vi "ReactionWheel.vi"(10 "Roll bias (deg)":dbl=0.5) -> ()   [LabVIEW 2021]
doc: "The myRIO Project template acquires acceleration data from the onboard accelerometer and displays the changes of acceleration values in a waveform chart."
uses:
  <vilib>/Platform/TimedLoop/XDataNode/timing_clust.ctl
  <vilib>/Platform/TimedLoop/XDataNode/nitl_modes.ctl
  <vilib>/Platform/TimedLoop/XDataNode/wakeup.ctl
  <vilib>/myRIO/Instrument Drivers/Onboard IO/PWM/typedefs/PWM Reference.ctl
  <vilib>/myRIO/Common/Instrument Driver Framework/Utilities/typedefs/myRIO Generic Hardware Reference.ctl
  <vilib>/myRIO/Common/Instrument Driver Framework/Utilities/typedefs/Hardware Version Enum.ctl
  <vilib>/myRIO/Common/Instrument Driver Framework/Utilities/typedefs/myRIO v1.0 Reference.ctl
  <vilib>/myRIO/Common/Instrument Driver Framework/Utilities/typedefs/Generic FPGA Reference.ctl
  <vilib>/myRIO/Common/Instrument Driver Framework/myRIO v1.0/PWM/typedefs/PWM Channels Enum.ctl
  <vilib>/myRIO/Instrument Drivers/Onboard IO/PWM/typedefs/PWM Configuration.ctl
  <vilib>/userdefined/High Color/nirio_resource_hc.ctl
  <vilib>/myRIO/Instrument Drivers/Onboard IO/UART/typedef/VISA Configuration.ctl
  <vilib>/myRIO/Common/Instrument Driver Framework/Utilities/vis/Is FPGA Ref Available.vi
  <vilib>/myRIO/Common/Instrument Driver Framework/myRIO v1.0/PWM/vis/myRIO v1.1 Open PWM.vi
  <vilib>/myRIO/Instrument Drivers/Onboard IO/PWM/vis/Set Duty Cycle and Frequency.vi
  <vilib>/myRIO/Common/Instrument Driver Framework/Utilities/vis/Validate Channels.vi
  <vilib>/myRIO/Common/Instrument Driver Framework/myRIO v1.0/PWM/vis/myRIO v1.0 Reserve PWM.vi
  <vilib>/myRIO/Common/Instrument Driver Framework/myRIO v1.0/PWM/vis/myRIO v1.0 Build MUX Configuration PWM.vi
  <vilib>/myRIO/Common/Instrument Driver Framework/myRIO v1.0/Resource Manager/vis/myRIO v1.0 Reserve Channel List.vi
  <vilib>/myRIO/Common/Instrument Driver Framework/myRIO v1.0/Resource Manager/vis/myRIO v1.0 Create Configuration List.vi
  <vilib>/myRIO/Common/Instrument Driver Framework/myRIO v1.0/Resource Manager/vis/myRIO v1.0 Reserve Channel.vi
  <vilib>/myRIO/Common/Instrument Driver Framework/myRIO v1.0/Resource Manager/vis/myRIO v1.0 Unreserve Channel.vi
  <vilib>/myRIO/Common/Instrument Driver Framework/myRIO v1.0/Resource Manager/vis/myRIO v1.0 Build Mutex Name.vi
  <vilib>/addons/control/pid/pid.llb/PID (DBL).vi
  <vilib>/Utility/VariantDataType/GetNumericInfo.vi
  <vilib>/Utility/error.llb/Error Cluster From Error Code.vi
  <vilib>/myRIO/Common/Instrument Driver Framework/myRIO v1.0/myRIO v1.1 Open.vi
  <vilib>/myRIO/Common/Instrument Driver Framework/Utilities/vis/IO Manager.vi
  <vilib>/myRIO/Common/Instrument Driver Framework/Utilities/vis/Configuration Manager.vi
  <vilib>/myRIO/Common/Instrument Driver Framework/myRIO v1.0/Resource Manager/vis/myRIO v1.0 Configure IO.vi
  <vilib>/myRIO/Common/Instrument Driver Framework/myRIO v1.0/myRIO v1.0 Close.vi
  <vilib>/myRIO/Common/Instrument Driver Framework/myRIO v1.0/PWM/vis/myRIO v1.0 Write PWM.vi
  <vilib>/Instr/_visa.llb/VISA Configure Serial Port (Instr).vi
  <vilib>/Platform/TimedLoop/XDataNode/XDataNode.xnode
  <vilib>/myRIO/Express VI/Onboard IO/PWM/PWM Express VI.xnode
  <vilib>/myRIO/Instrument Drivers/Onboard IO/PWM/vis/myRIO PWM Open.xnode
  <vilib>/myRIO/Express VI/Onboard IO/UART/UART Express VI.xnode
  <vilib>/myRIO/Instrument Drivers/Onboard IO/UART/UART.lvlib
  <vilib>/Platform/TimedLoop/XDataNode/XDNodeRunTimeDep.lvlib
  <vilib>/myRIO/Instrument Drivers/Onboard IO/PWM/PWM.lvlib
  <vilib>/addons/control/pid/NI_PID_pid.lvlib
panel:
  out "Ref. error":dbl
  out "Roll reference":dbl
  out "Roll (deg)":dbl
  in  "Visualisation period (ms)":dbl=250.0
  out "PID error out":errorcluster
  in  "PWMfrekvens":dbl=4000.0
  in  "PID output range":cluster{"Maximum":dbl, "Minimum":dbl}={"Maximum"=0.25, "Minimum"=-0.25}
  in  "PID gains":cluster{"P":dbl, "I":dbl, "D":dbl}
  in  "UART read period (ms)":dbl=25.0
  out "UART error out":errorcluster
  in  "PID period (ms)":dbl=100.0
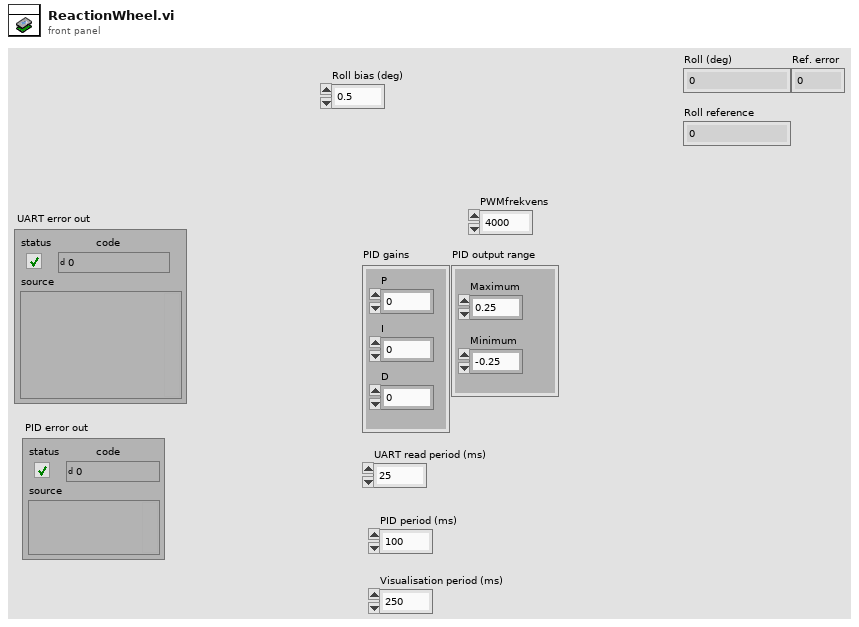
[diagram p1: front panel]
types:
  T1 = cluster{"Roll (deg)":dbl, "Roll reference":dbl, "PID output":dbl}
  T2 = typedef "XDNodeRunTimeDep.lvlib/timing_clust.ctl" = cluster{"Expected End [f-1]":u64, "Actual End [f-1]":u64, "Finished Late? [f-1]":bool, "Expected End [i-1]":u64, "Actual End [i-1]":u64, "Finished Late? [i-1]":bool, "Expected Start [i]":u64, "Actual Start [i]":u64, "Expected Start [f]":u64, "Actual Start [f]":u64, "Source Name":string, "Structure Name":string, "Period":i64, "Deadline":i64, "Offset":i64, "Start":i64, "Priority":i32, "Timeout":i32, "Mode":T3, "Wakeup Reason":T4, "Error":errorcluster, "Source Type":string, "Secondary Source Type":string, "Global End Time":u64, "Global Start Time":u64, "Frame Duration":u64, "Iteration Duration":u64, "Assigned CPU":i32, "I/O Scan Engine Mode":u32}
  T3 = typedef "XDNodeRunTimeDep.lvlib/nitl_modes.ctl" = enum32{"No Change", "Process missed periods, maintain original phase", "Discard missed periods, maintain original phase", "Process missed periods, ignore original phase", "Discard missed periods, ignore original phase"}
  T4 = typedef "XDNodeRunTimeDep.lvlib/wakeup.ctl" = enum32{"Normal", "Aborted", "Asynchronous wakeup", "Timing source error", "Timed loop error", "Timeout"}
  T5 = typedef "UART.lvlib/VISA Configuration.ctl" = cluster{"baud rate (9600)":u32, "data bits (8)":u16, "parity (0:none)":enum16{"None", "Odd", "Even", "Mark", "Space"}, "stop bits (10: 1 bit)":u16, "flow control (0:none)":u16, "termination char\n(0xA = '\\n' = LF) ":u8, "Enable Termination\nChar (T)":bool, "timeout (10sec)":u32}
  T6 = typedef "PWM.lvlib/PWM Reference.ctl" = cluster{"myRIO Reference":T7, "PWM Channels Enum":T11, "PWM Configuration":T12}
  T7 = typedef "myRIO Generic Hardware Reference.ctl" = cluster{"myRIO Model":T8, "myRIO Hardware Reference":T9}
  T8 = typedef "Hardware Version Enum.ctl" = enum16{"Unknown", "myRIO-1900", "myRIO-1950", "roboRIO", "NI ELVIS RIO CM", "ELVIS III"}
  T9 = typedef "myRIO v1.0 Reference.ctl" = cluster{"Generic FPGA Reference":T10, "Allow multiple opens":bool}
  T10 = typedef "Generic FPGA Reference.ctl" = refnum<k20>
  T11 = typedef "PWM Channels Enum.ctl" = enum16{"Not Connected", "C/PWM0", "C/PWM1", "A/PWM0", "A/PWM1", "A/PWM2", "A/PWM3", "A/PWM4", "A/PWM5", "A/PWM6", "A/PWM7", "A/PWM8", "A/PWM9", "A/PWM10", "A/PWM11", "A/PWM12", "A/PWM13", "A/PWM14", "A/PWM15", "A/PWM16", "A/PWM17", "A/PWM18", "A/PWM19", "B/PWM0", "B/PWM1", "B/PWM2", "B/PWM3", "B/PWM4", "B/PWM5", "B/PWM6", "B/PWM7", "B/PWM8", "B/PWM9", "B/PWM10", "B/PWM11", "B/PWM12", "B/PWM13", "B/PWM14", "B/PWM15", "B/PWM16", "B/PWM17", "B/PWM18", "B/PWM19", "PWM/PWM0", "PWM/PWM1", "PWM/PWM2", "PWM/PWM3", "PWM/PWM4", "PWM/PWM5", "PWM/PWM6", "PWM/PWM7", "PWM/PWM8", "PWM/PWM9"}
  T12 = typedef "PWM.lvlib/PWM Configuration.ctl" = cluster{"Frequency":dbl, "Duty Cycle":dbl}
  T13 = typedef "nirio_resource_hc.ctl" = tag
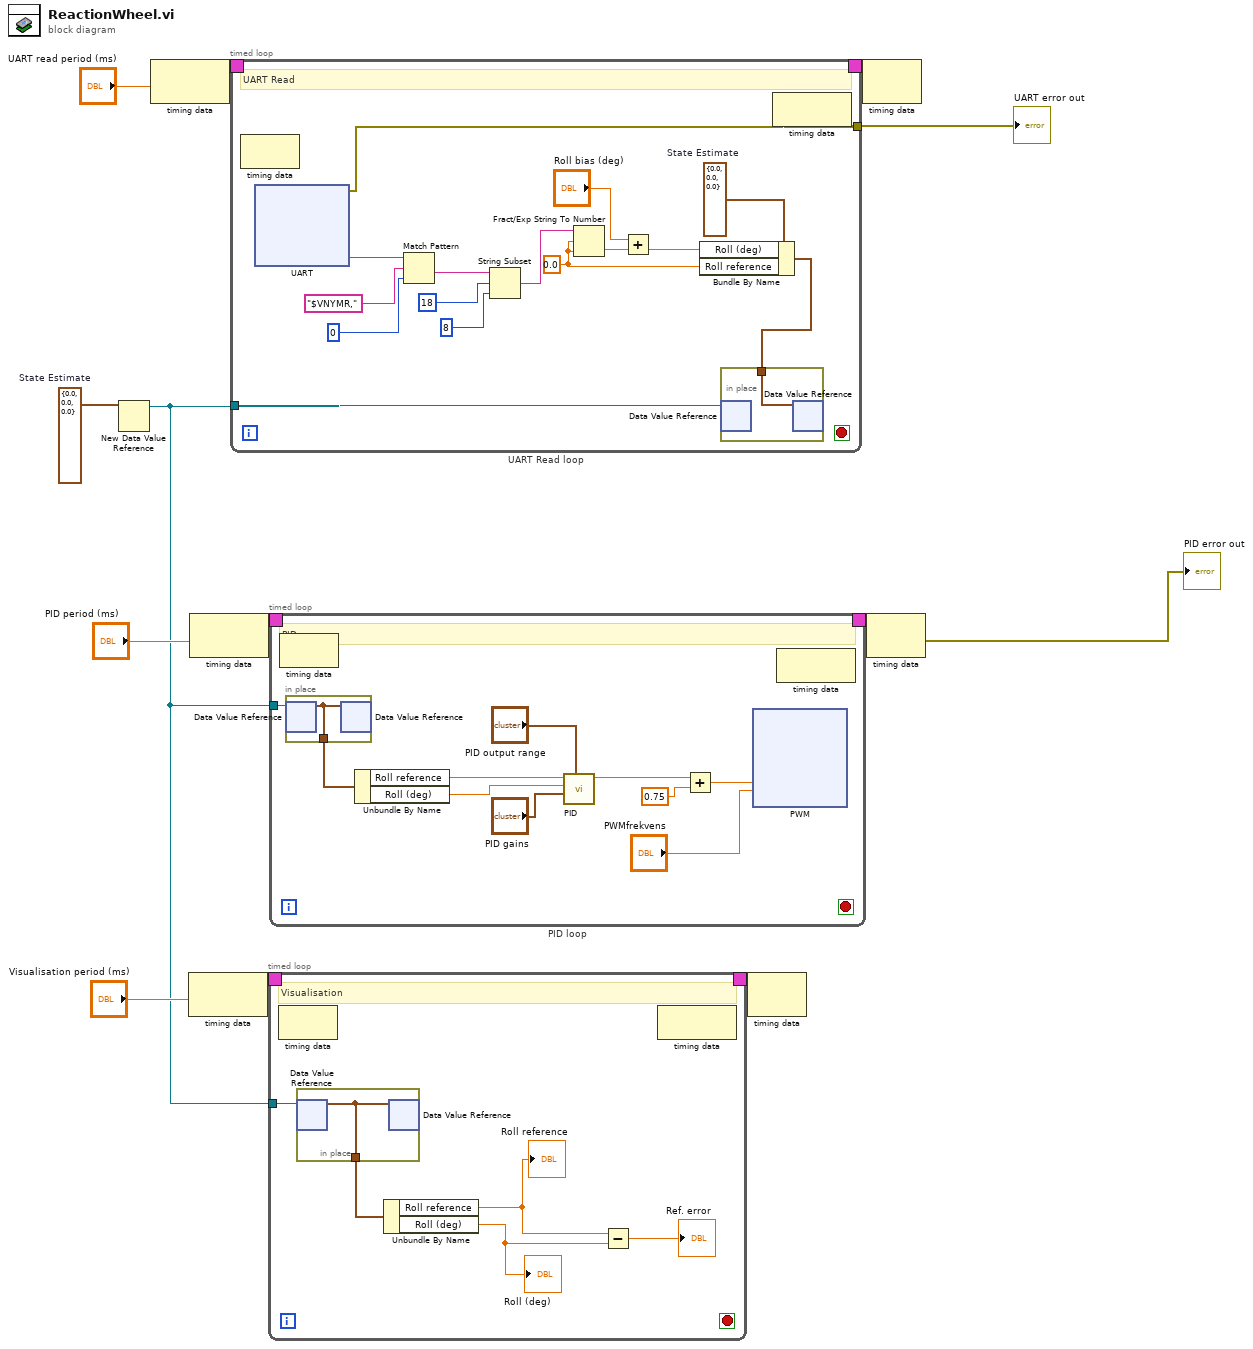
[diagram p0: block diagram]
diagram:
  w6 = T1 {"Roll (deg)"=0.0, "Roll reference"=0.0, "PID output"=0.0}  # State Estimate
  n1 = New Data Value Reference(data value=w6) -> (data value reference=w1:refnum<data-value>)  [unwired: 1 in, 1 out]
  n2 = node-c288("UART read period (ms)") -> (w13:T2)
  n3 = node-c288("Visualisation period (ms)") -> (w4:T2)
  n4 = node-c288("PID period (ms)") -> (w11:T2)
  n5 = timed-loop "UART Read loop" {
    timing: w13 -> [_]
    timing-out: [_] -> w12
    tunnel: [w22] -> w9
    tunnel: w1 -> [w20]
    stop <- _ stop-if-true
    w18 = T1 {"Roll (deg)"=0.0, "Roll reference"=0.0, "PID output"=0.0}  # State Estimate
    w16 = 0.0
    # "UART Read"
    n6 = node-c288() -> ()  [unwired: 1 in, 1 out]
    n7 = xnode "UART"() -> ("Characters Read"=w28:string, "error out"=w22:errorcluster)  [unwired: 1 in]
    n8 = Match Pattern(string=w28, regular expression="$VNYMR,", offset (0)=0) -> (after substring=w27:string)  [unwired: 3 out]
    n9 = String Subset(string=w27, offset (0)=18, length (rest)=8) -> (substring=w21:string)
    n10 = Fract/Exp String To Number(string=w21, offset=w16, default (0 dbl)=w16) -> (number=w17:dbl)  [unwired: 1 in, 1 out]
    n11 = Add(x="Roll bias (deg)", y=w17) -> (x+y=w15:dbl)
    n12 = Bundle By Name(cluster=w18, "Roll (deg)"=w15, "Roll reference"=w16) -> (w19:T1)
    n13 = in-place {
      in-place-border: w19 -> [w29]
      n14 = in-place-dvr #1(w20) -> ()  [unwired: 2 out]
      n15 = in-place-dvr #1(w29) -> ()  [unwired: 2 out]
    }
    n16 = node-c288() -> ()  [unwired: 1 in, 1 out]
  }
  "UART error out" <- w9
  n17 = timed-loop {
    timing: w4 -> [_]
    timing-out: [_] -> w3
    tunnel: w1 -> [w53]
    stop <- _ stop-if-true
    # "Visualisation"
    n18 = node-c288() -> ()  [unwired: 1 in, 1 out]
    n19 = in-place {
      in-place-border: [w54] -> w52
      n20 = in-place-dvr #2(w53) -> (w54:T1)  [unwired: 1 out]
      n21 = in-place-dvr #2(w54) -> ()  [unwired: 2 out]
    }
    n22 = Unbundle By Name(w52) -> ("Roll reference"=w50:dbl, "Roll (deg)"=w49:dbl)
    "Roll (deg)" <- w49
    "Roll reference" <- w50
    n23 = Subtract(x=w50, y=w49) -> (x-y=→"Ref. error":dbl)
    n24 = node-c288() -> ()  [unwired: 1 in, 1 out]
  }
  n25 = timed-loop "PID loop" {
    timing: w11 -> [_]
    timing-out: [_] -> w10
    tunnel: w1 -> [w62]
    stop <- _ stop-if-true
    # "PID"
    n26 = node-c288() -> ()  [unwired: 1 in, 1 out]
    n27 = in-place {
      in-place-border: [w67] -> w60
      n28 = in-place-dvr #3(w62) -> (w67:T1)  [unwired: 1 out]
      n29 = in-place-dvr #3(w67) -> ()  [unwired: 2 out]
    }
    n30 = Unbundle By Name(w60) -> ("Roll reference"=w59:dbl, "Roll (deg)"=w61:dbl)
    n31 = call-poly <vilib>:"PID.vi"("output range"="PID output range", "PID gains"="PID gains", "process variable"=w61, "setpoint"=w59) -> ("output"=w57:dbl)  [unwired: 6 in, 1 out]
    n32 = Add(x=w57, y=0.75) -> (x+y=w64:dbl)
    n33 = xnode "PWM"("Duty Cycle"=w64, "Frequency [Hz]"="PWMfrekvens") -> ()  [unwired: 1 in, 1 out]
    n34 = node-c288() -> ()  [unwired: 1 in, 1 out]
  }
  n35 = node-c288(w3) -> ()  [unwired: 1 out]
  n36 = node-c288(w12) -> ()  [unwired: 1 out]
  n37 = node-c288(w10) -> (→"PID error out":errorcluster)
